vi "Read DC Power.vi"(8 "error in (no error)":errorcluster, 11 "LTB-1 in":refnum<class "LTB-1.lvclass">) -> (0 "error out":errorcluster, 2 "Power (uW)":dbl, 3 "LTB-1 out":refnum<class "LTB-1.lvclass">, 4 "Power (dBm)":dbl)   [LabVIEW 2018, in "LTB-1.lvlib" / "LTB-1.lvclass"]
doc: "This is a dynamically dispatched VI. The child class will return the power levels in microWatts measured by the variable optical attenuator. VOA Power meter reports in dB - use appropriate equations to convert from dB to uW.\n\nAuthor: Ron Dexter\nCompany: Luminar\nModified: 5/20/2018"
uses:
  LTB-1.lvclass
  C:/AME Test Engineering/LabVIEW/PPLs/EXFO/Parent/EXFO.lvlibp/EXFO.lvclass
  LTB-1.lvclass/LTB-1.ctl
  PPLs/EXFO/Parent/EXFO.lvlibp/Methods/Read Resource.vi
  3150 Driver/3150.lvlib
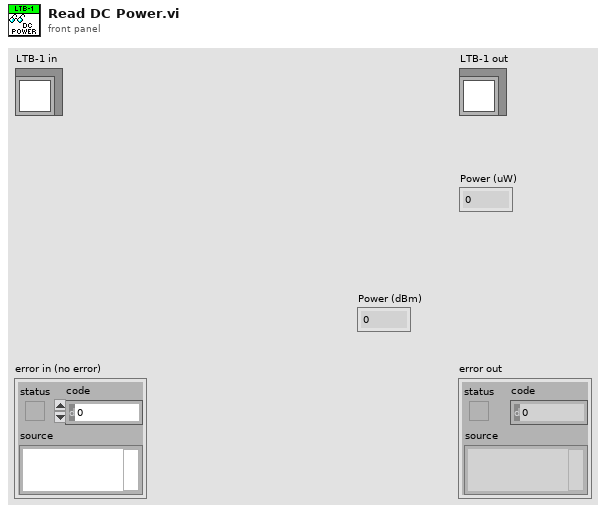
[diagram p1: front panel]
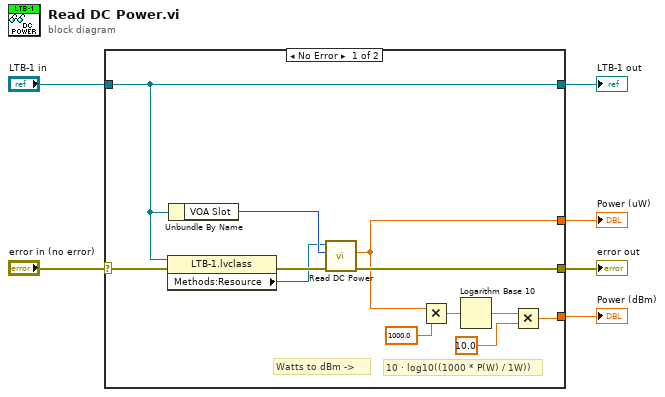
[diagram p0: block diagram]
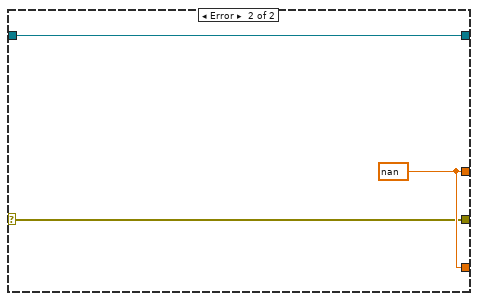
[diagram p2: hidden frame]
diagram:
  n1 = case shown="No Error" "error in (no error)" {
    selector: "error in (no error)" -> [w18 w19]
    tunnel: "LTB-1 in" -> [w17 w21]
    tunnel: [w7 w20] -> w4
    tunnel: [w17 w21] -> w3
    tunnel: [w12 w20] -> w2
    tunnel: [w10 w19] -> w1
    frame No Error {
      # "Watts to dBm ->"
      # "10 · log10((1000 * P(W) / 1W))"
      n2 = property class="LTB-1.lvclass"(reference=w17, error in=w18) -> (error out=w11:errorcluster, "Methods:Resource"=w8:refnum<visa-resource-name>)  [unwired: 1 out]
      n3 = Unbundle By Name(w17) -> ("VOA Slot"=w9:i16)
      n4 = call "Read DC Power.vi"("error in (no error)"=w11, "Platform Slot Number (10)"=w9, "VISA resource name"=w8) -> ("error out"=w10:errorcluster, "Power Measurement"=w7:dbl)  [unwired: 6 in, 1 out]
      n5 = Multiply(x=w7, y=1000.0) -> (x*y=w14:dbl)
      n6 = Logarithm Base 10(1:w14) -> (0:w13:dbl)
      n7 = Multiply(x=w13, y=10.0) -> (x*y=w12:dbl)
    }
    frame Error {
      w20 = nan ("Output Power")
    }
  }
  "error out" <- w1
  "LTB-1 out" <- w3
  "Power (uW)" <- w4
  "Power (dBm)" <- w2
